vi "init.vi"() -> (0 "error out":errorcluster, 3 "Modules":T1)   [LabVIEW 2025]
uses:
  <vilib>/Utility/sysdir.llb/System Directory Type.ctl
  Libraries/USB IO/Classes/Hardware Selection.ctl
  Libraries/USB IO/USB IO.lvlib
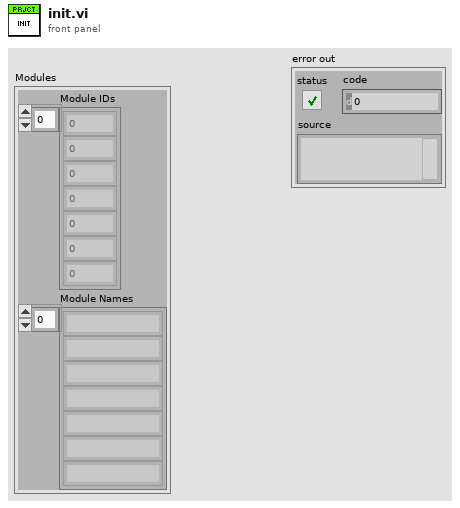
[diagram p1: front panel]
types:
  T1 = cluster{"Module IDs":i32[], "Module Names":string[]}
  T2 = typedef "Hardware Selection.ctl" = enum16{"Simulation", "USB-6000", "USB-6001", "Arduino Uno"}
  T3 = typedef "System Directory Type.ctl" = i32
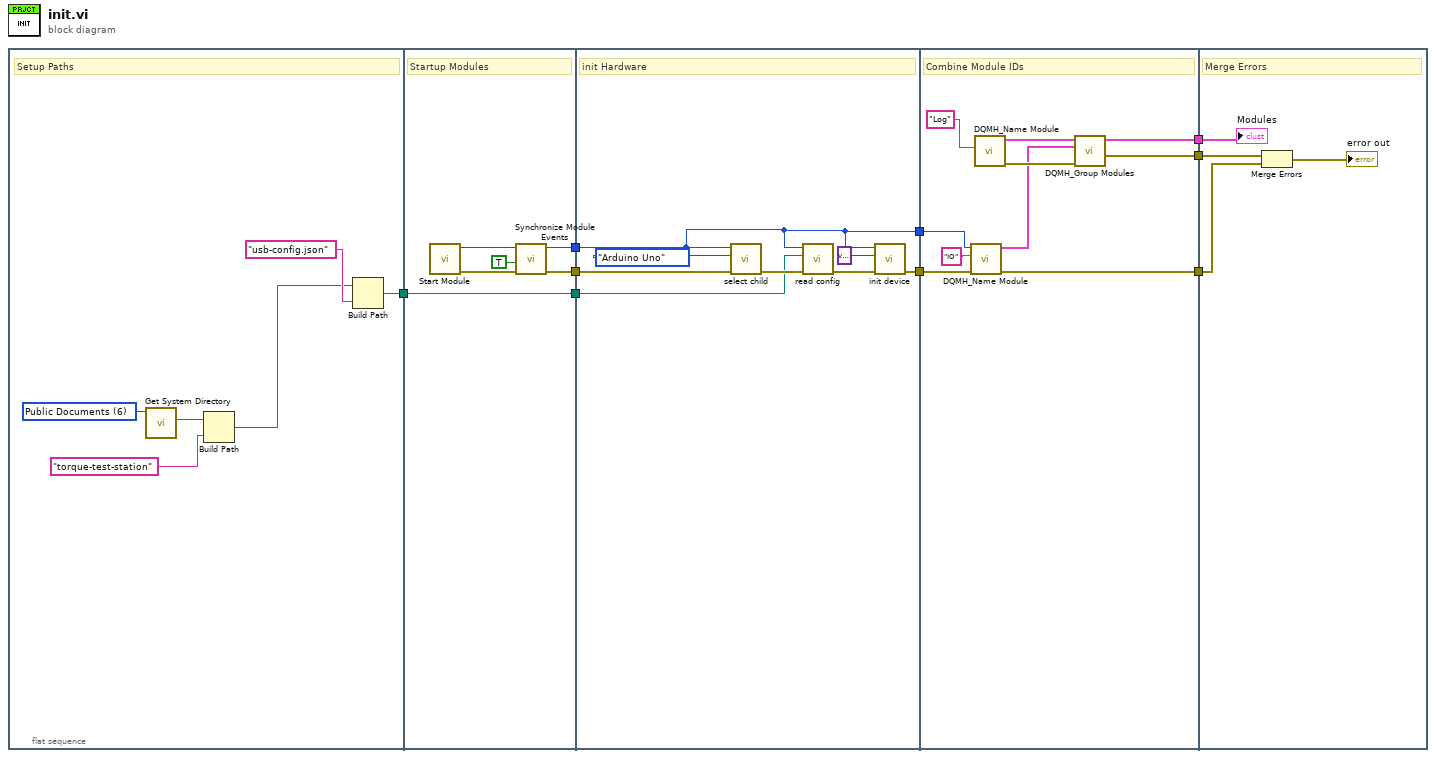
[diagram p0: block diagram]
diagram:
  n1 = flat-sequence {
    tunnel: [w10] -> w5
    tunnel: [w18] -> w7
    tunnel: [w17] -> w6
    tunnel: w5 -> [w16]
    tunnel: [w16] -> w4
    tunnel: w7 -> [w23]
    tunnel: w6 -> [w29]
    tunnel: w4 -> [w26]
    tunnel: [w23] -> w3
    tunnel: [w22] -> w2
    tunnel: [w36] -> w9
    tunnel: [w35] -> w8
    tunnel: w3 -> [w34]
    tunnel: w2 -> [w32]
    tunnel: [w30] -> w1
    tunnel: w9 -> [w42]
    tunnel: w8 -> [w43]
    tunnel: w1 -> [w40]
    frame #0 {
      w15 = T3 6 items=["User Home"=0, "User Desktop"=1, "User Documents"=2, "User Application Data"=3, "User Preferences"=4, "User Temporary"=5, "Public Documents"=6, "Public Application Data"=7, "Public Preferences"=8, "Public Cache"=13, "System Core Libraries"=9, "System Installed Libraries"=10, "Application Files"=11, "Boot Volume Root"=12] ("system directory type")
      # "Setup Paths"
      n2 = call <vilib>:"Get System Directory.vi"("system directory type"=w15) -> ("system directory"=w14:path)  [unwired: 10 in]
      n3 = Build Path(base path=w14, name or relative path="torque-test-station") -> (appended path=w11:path)
      n4 = Build Path(base path=w11, name or relative path="usb-config.json") -> (appended path=w10:path)
    }
    frame #1 {
      # "Startup Modules"
      n5 = call "Start Module.vi"() -> ("error out"=w20:errorcluster, "Module ID"=w21:i32)  [unwired: 7 in, 3 out]
      n6 = call "Synchronize Module Events.vi"("error in"=w20, "Wait for Event Sync?"=TRUE, "Module ID in"=w21) -> ("error out"=w17:errorcluster, "Module ID out"=w18:i32)  [unwired: 7 in]
    }
    frame #2 {
      # "init Hardware"
      n7 = call "select child.vi"("error in"=w29, "Hardware"=Hardware_Selection."Arduino Uno", "Module ID"=w23) -> ("error out"=w27:errorcluster)  [unwired: 7 in, 1 out]
      n8 = call "read config.vi"("error in"=w27, "Path"=w26, "Module ID"=w23) -> ("error out"=w25:errorcluster)  [unwired: 7 in, 1 out]
      n9 = call "init device.vi"("error in"=w25, "Variant"=variant, "Module ID"=w23) -> ("error out"=w22:errorcluster)  [unwired: 7 in, 1 out]
    }
    frame #3 {
      # "Combine Module IDs"
      n10 = call "DQMH_Name Module.vi"("error in"=w32, "String"="IO", "Module ID in"=w34) -> ("error out"=w30:errorcluster, "input cluster"=w31:T1)  [unwired: 7 in]
      n11 = call "DQMH_Name Module.vi"("String"="Log") -> ("error out"=w37:errorcluster, "input cluster"=w38:T1)  [unwired: 9 in]
      n12 = call "DQMH_Group Modules.vi"("error in (no error)"=w37, "Module 2"=w31, "Module 1"=w38) -> ("error out"=w36:errorcluster, "Modules"=w35:T1)  [unwired: 7 in]
    }
    frame #4 {
      # "Merge Errors"
      n13 = Merge Errors(w42, w40) -> (→"error out":errorcluster)
      "Modules" <- w43
    }
  }
